vi "Read Data String.vi"(8 "error in (no error)":errorcluster, 11 "Project Builder in":refnum<class "Project Builder.lvclass">) -> (0 "error out":errorcluster, 2 "Data":string, 3 "Project Builder out":refnum<class "Project Builder.lvclass">)   [LabVIEW 2019, in "ProjectBuilder.lvlib" / "Project Builder.lvclass"]
uses:
  Project Builder.lvclass
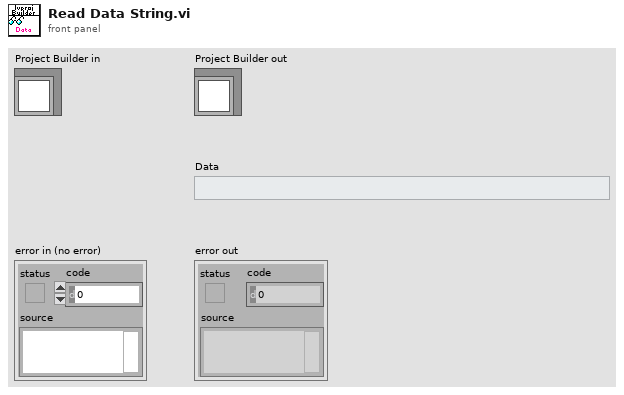
[diagram p1: front panel]
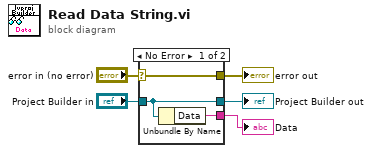
[diagram p0: block diagram]
diagram:
  n1 = case shown="No Error" "error in (no error)" {
    selector: "error in (no error)" -> [w8 w9]
    tunnel: [w8 w9] -> w4
    tunnel: [w7 w10] -> w2
    tunnel: "Project Builder in" -> [w7 w10]
    tunnel: [w6 _] -> w1
    frame No Error {
      n2 = Unbundle By Name(w7) -> ("Data"=w6:string)
    }
    frame Error {
    }
  }
  "error out" <- w4
  "Project Builder out" <- w2
  "Data" <- w1
